vi "Stem-and-Leaf Plot.vi"(9 "Precision (6)":i16=2, 10 "Number of divisions":u8=14 min=1, 11 "Data array":dbl[](array[numeric]) format="%#.6g") -> (3 "Stem-and-Leaf Display":string)   [LabVIEW 2023]
doc: "Creates a stem-and-leaf display of the data."
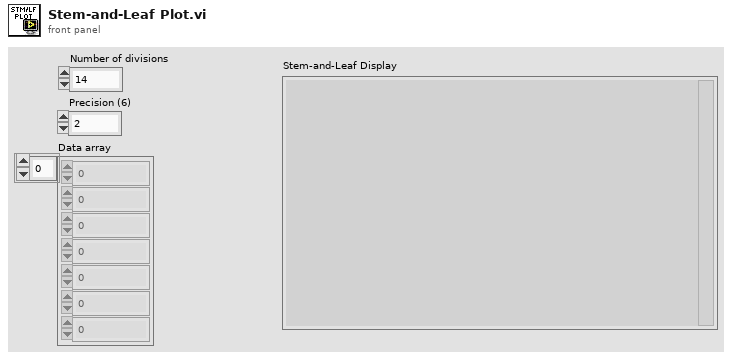
[diagram p1: front panel]
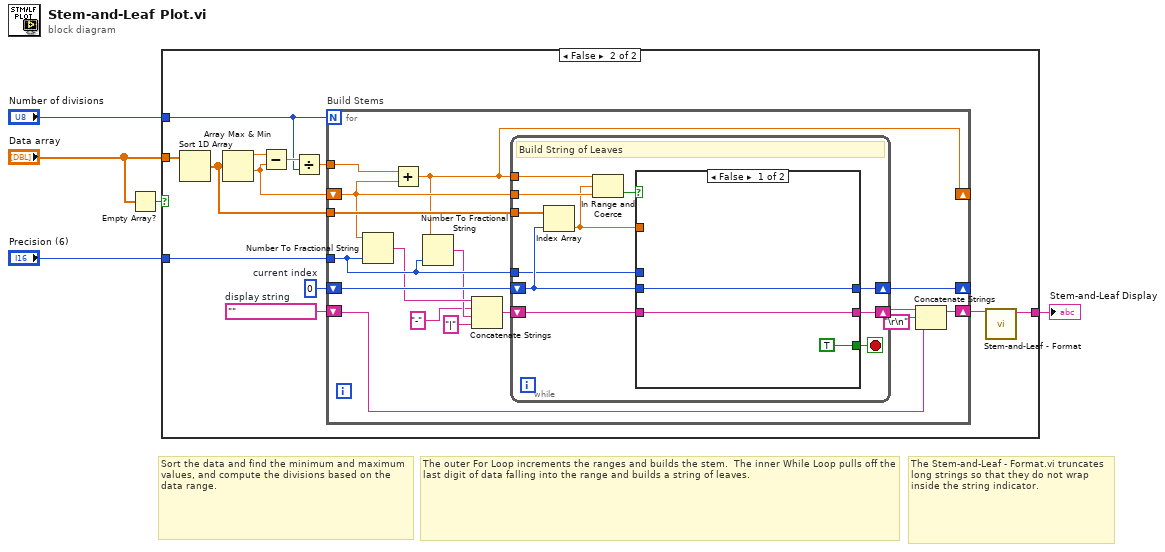
[diagram p0: block diagram]
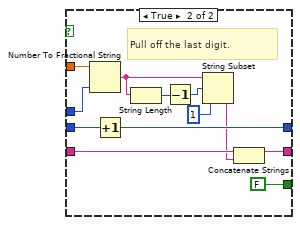
[diagram p3: hidden frame]
diagram:
  # "The Stem-and-Leaf - Format.vi truncates long strings so that they do not wrap inside the string indicator."
  # "The outer For Loop increments the ranges and builds the stem.  The inner While Loop pulls off the last digit of data falling into the range and builds a string of leaves."
  # "Sort the data and find the minimum and maximum values, and compute the divisions based on the data range."
  n1 = Empty Array?(array="Data array") -> (empty?=w1:bool)
  n2 = case shown="False" w1 {
    tunnel: "Data array" -> [_ w13]
    tunnel: [_ w8] -> w5
    tunnel: "Number of divisions" -> [_ w7]
    tunnel: "Precision (6)" -> [_ w6]
    frame True {
      # "Array is empty so do nothing"
    }
    frame False {
      w11 = ""  # display string
      w17 = 0  # current index
      n3 = Sort 1D Array(array=w13) -> (sorted array=w10:dbl[])
      n4 = Array Max & Min(array=w10) -> (max value=w14:dbl, min value=w15:dbl)  [unwired: 2 out]
      n5 = Subtract(x=w14, y=w15) -> (x-y=w16:dbl)
      n6 = Divide(x=w16, y=w7) -> (x/y=w12:dbl)
      n7 = for "Build Stems" {
        N: w7 -> [_]
        tunnel: w12 -> [w26]
        tunnel: w10 -> [w28]
        shift-right: [w32] -> _
        shift-left: w17 -> [w33]
        shift-right: [w25] -> _
        shift-left: w15 -> [w27]
        shift-right: [w30] -> w9
        shift-left: w11 -> [w23]
        tunnel: w6 -> [w24]
        n8 = Number To Fractional String(number=w27, precision (6)=w24) -> (F-format string=w22:string)  [unwired: 2 in]
        n9 = Add(x=w26, y=w27) -> (x+y=w25:dbl)
        n10 = Number To Fractional String(number=w25, precision (6)=w24) -> (F-format string=w20:string)  [unwired: 2 in]
        n11 = Concatenate Strings(w22, "-" ("string"), w20, "|" ("string")) -> (w19:string)
        n12 = while {
          shift-right: [w40] -> w32
          shift-left: w33 -> [w41]
          tunnel: w28 -> [w44]
          tunnel: w27 -> [w39]
          tunnel: w25 -> [w38]
          shift-right: [w35] -> w31
          shift-left: w19 -> [w36]
          tunnel: w24 -> [w34]
          stop <- w42 stop-if-true
          # "Build String of Leaves"
          n13 = Index Array(array=w44, index=w41) -> (element=w37:dbl)
          n14 = In Range and Coerce(upper limit=w38, x=w37, lower limit=w39) -> (In Range?=w43:bool)  [unwired: 1 out]
          n15 = case shown="False" w43 {
            tunnel: [TRUE FALSE] -> w42
            tunnel: w41 -> [w47 w58]
            tunnel: [w47 w57] -> w40
            tunnel: w37 -> [_ w56]
            tunnel: w36 -> [w45 w52]
            tunnel: [w45 w51] -> w35
            tunnel: w34 -> [_ w50]
            frame False {
            }
            frame True {
              # "Pull off the last digit."
              n16 = Number To Fractional String(number=w56, precision (6)=w50) -> (F-format string=w55:string)  [unwired: 2 in]
              n17 = Increment(x=w58) -> (x+1=w57:i32)
              n18 = String Length(string=w55) -> (length=w48:i32)
              n19 = Decrement(x=w48) -> (x-1=w53:i32)
              n20 = String Subset(string=w55, offset (0)=w53, length (rest)=1 ("y")) -> (substring=w49:string)
              n21 = Concatenate Strings(w52, w49) -> (w51:string)
            }
          }
        }
        n22 = Concatenate Strings(w31, "\r\n", w23) -> (w30:string)
      }
      n23 = call "Stem-and-Leaf - Format.vi"("String In"=w9) -> ("String Formatted"=w8:string)  [unwired: 10 in]
    }
  }
  "Stem-and-Leaf Display" <- w5
